vi "ARM ROBOT.vi"() -> ()   [LabVIEW 2019]
uses:
  <vilib>/Instr/_visa.llb/VISA Configure Serial Port (Instr).vi
panel:
  in  "Boolean":bool
  out "error out":errorcluster
  in  "VISA resource name":refnum<visa-resource-name>
  in  "stop":bool
  out "Baca Serial":string
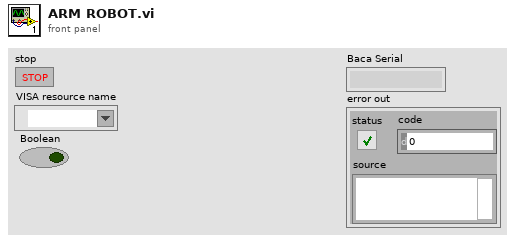
[diagram p1: front panel]
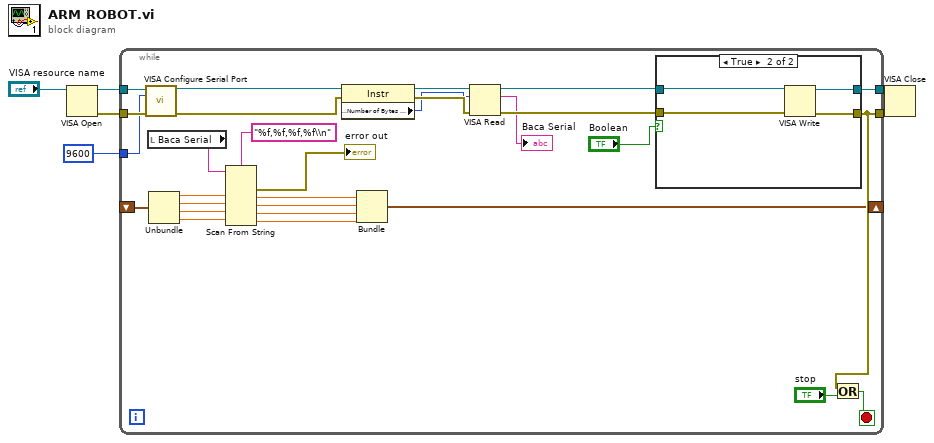
[diagram p0: block diagram]
diagram:
  n1 = VISA Open(VISA resource name="VISA resource name") -> (VISA resource name=w6:refnum<visa-resource-name>, error out=w5:errorcluster)  [unwired: 4 in]
  n2 = while {
    tunnel: w6 -> [w30]
    tunnel: [w26] -> w4
    tunnel: w5 -> [w29]
    tunnel: [w22] -> w3
    tunnel: u32 9600 ("baud rate (9600)") -> [w21]
    shift-right: [w14] -> _
    shift-left: _ -> [w13]
    stop <- w23 stop-if-true
    n3 = call-poly "VISA Configure Serial Port"("VISA resource name"=w30, "baud rate (9600)"=w21, "error in (no error)"=w29) -> ("VISA resource name out"=w33:refnum<visa-resource-name>, "error out"=w32:errorcluster)  [unwired: 11 in]
    n4 = local read "Baca Serial"() -> (w20:string)
    n5 = Unbundle(w13) -> (w12:dbl, w11:dbl, w10:dbl, w9:dbl)
    n6 = Scan From String(format string="%f,%f,%f,%f\\n", input string=w20, default 1=w12, default 2=w11, default 3=w10, default 4=w9) -> (error out=→"error out":errorcluster, output 1=w18:dbl, output 2=w17:dbl, output 3=w16:dbl, output 4=w15:dbl)  [unwired: 2 in, 2 out]
    n7 = property class="Instr"(reference=w33, error in=w32) -> (reference out=w35:refnum<visa-resource-name>, error out=w34:errorcluster, "Serial Settings:Number of Bytes at Serial Port"=w31:u32)
    n8 = Bundle(w18, w17, w16, w15) -> (w14:cluster{dbl, dbl, dbl, dbl})  [unwired: 1 in]
    n9 = VISA Read(VISA resource name=w35, byte count=w31, error in (no error)=w34) -> (VISA resource name out=w28:refnum<visa-resource-name>, read buffer=→"Baca Serial":string, error out=w27:errorcluster)  [unwired: 1 out]
    n10 = case shown="True" "Boolean" {
      tunnel: w28 -> [w37 w41]
      tunnel: w27 -> [w36 w40]
      tunnel: [w37 w39] -> w26
      tunnel: [w36 w38] -> w22
      frame False {
      }
      frame True {
        n11 = VISA Write(VISA resource name=w41, error in (no error)=w40) -> (VISA resource name out=w39:refnum<visa-resource-name>, error out=w38:errorcluster)  [unwired: 1 in, 1 out]
      }
    }
    n12 = Or(x=w22, y="stop") -> (x .or. y?=w23:bool)
  }
  n13 = VISA Close(VISA resource name=w4, error in (no error)=w3) -> ()  [unwired: 1 out]
